vi "lvssh2_session_callback_register_kbdint_response_32.vi"(11 "keyboard-interactive response":refnum<vi>) -> (0 "error out":errorcluster, 2 "stop event":refnum<user-event>, 3 "user event":refnum<user-event>)   [LabVIEW 2017, in "libssh2.lvlib"]
uses:
  libssh2.lvlib
  lvssh2_userauth_keyboard_interactive_response_function_input_args_32.ctl
  lvssh2_userauth_keyboard_interactive_response_function_handler_32.vi
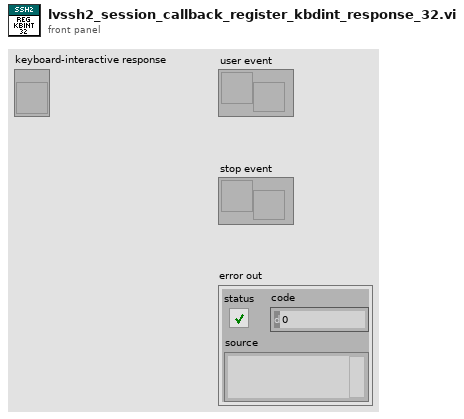
[diagram p1: front panel]
types:
  T1 = typedef "libssh2.lvlib/lvssh2_userauth_keyboard_interactive_response_function_input_args_32.ctl" = cluster{"name":string, "instruction":string, "num_prompts":i32, "*prompts":u32, "*responses":u32, "completion":u32}
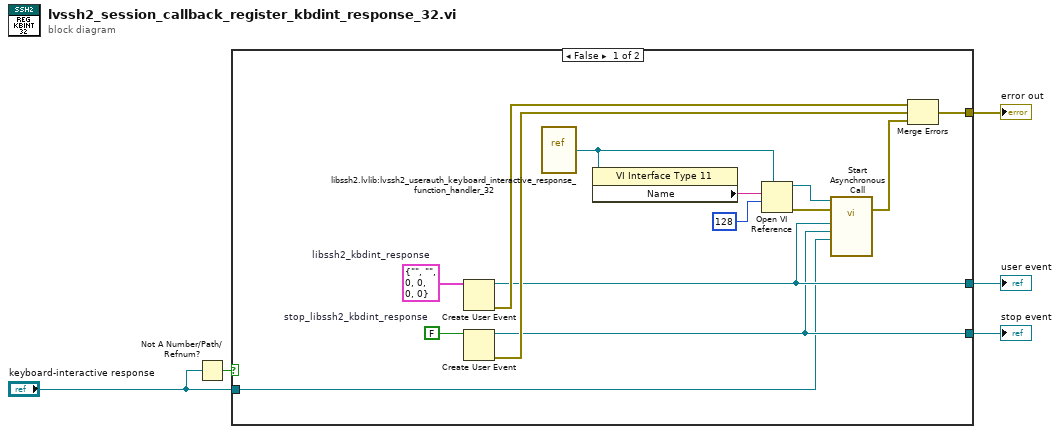
[diagram p0: block diagram]
diagram:
  n1 = Not A Number/Path/Refnum?(number/path/refnum="keyboard-interactive response") -> (NaN/Path/Refnum?=w3:bool)
  n2 = case shown="False" w3 {
    tunnel: [w8 _] -> w5
    tunnel: [w7 _] -> w1
    tunnel: [w19 _] -> w4
    tunnel: "keyboard-interactive response" -> [w6 _]
    frame False {
      w12 = FALSE  # stop_libssh2_kbdint_response
      w18 = T1 {"name"="", "instruction"="", "num_prompts"=0, "*prompts"=0, "*responses"=0, "completion"=0}  # libssh2_kbdint_response
      n3 = Create User Event(user event datatype=w18) -> (user event=w8:refnum<user-event>, error out=w17:errorcluster)  [unwired: 1 in]
      n4 = Create User Event(user event datatype=w12) -> (user event=w7:refnum<user-event>, error out=w10:errorcluster)  [unwired: 1 in]
      n5 = vi-ref "libssh2.lvlib:lvssh2_userauth_keyboard_interactive_response_function_handler_32.vi"() -> ("vi reference"=w11:refnum<vi>)
      n6 = property class="VI Interface Type 11"(reference=w11) -> ("Name"=w16:string)  [unwired: 1 in, 2 out]
      n7 = Open VI Reference(type specifier VI Refnum (for type only)=w11, vi path=w16, options=128) -> (vi reference=w13:refnum<vi>, error out=w14:errorcluster)  [unwired: 3 in]
      n8 = call-by-ref "Start Asynchronous Call"(reference=w13, error in=w14, "lvssh2_userauth_keyboard_interactive_response_function"=w6, "Stop Event Ref"=w7, "User Event Ref"=w8) -> (error out=w9:errorcluster)  [unwired: 9 in, 1 out]
      n9 = Merge Errors(w17, w10, w9) -> (w19:errorcluster)
    }
    frame True {
    }
  }
  "user event" <- w5
  "error out" <- w4
  "stop event" <- w1
